vi "Default Selector (Double).vi"(9 "Null Input":dbl, 10 "Default Value":dbl, 11 "Input Value":dbl) -> (3 "Output Value":dbl)   [LabVIEW 2015]
panel:
  # "Inputs"
  # "Outputs"
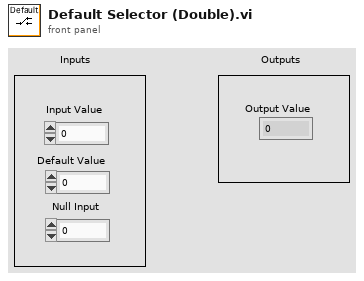
[diagram p1: front panel]
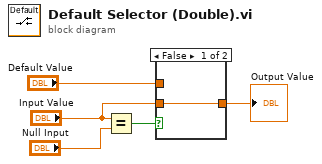
[diagram p0: block diagram]
diagram:
  n1 = Equal?(x="Input Value", y="Null Input") -> (x = y?=w5:bool)
  n2 = case shown="False" w5 {
    tunnel: "Input Value" -> [w6 _]
    tunnel: [w6 w7] -> w1
    tunnel: "Default Value" -> [_ w7]
    frame False {
    }
    frame True {
    }
  }
  "Output Value" <- w1
